vi "Check For Hardlink.vi"(8 "Error In":errorcluster, 10 "File Path":path, 11 "Configuration":T1) -> (0 "Error Out":errorcluster, 1 "Multiple Hardlinks":bool, 2 "Dup File Path":path, 3 "Configuration":T1)   [LabVIEW 2011, in "LVH-Toolbox.lvlib" / "LVH-Build-Tools.lvlib"]
uses:
  LVH-Build-Tools.lvlib
  Type Defs/Configuration.ctl
  Type Defs/Install Configuration.ctl
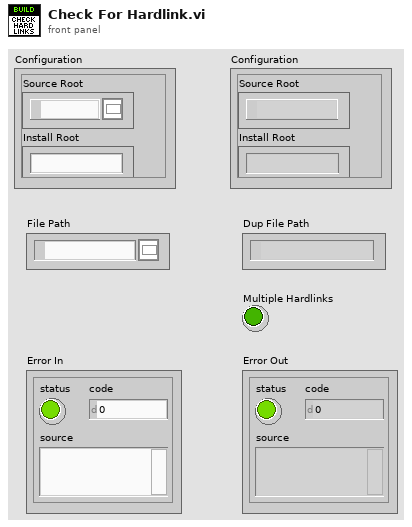
[diagram p1: front panel]
types:
  T1 = typedef "LVH-Toolbox.lvlib/LVH-Build-Tools.lvlib/Configuration.ctl" = cluster{"Source Root":path, "Install Root":string, "Components":string[], "Ignore":string[], "Config Files":path[], "LV Directories":path[], "Install Paths":T2}
  T2 = typedef "LVH-Toolbox.lvlib/LVH-Build-Tools.lvlib/Install Configuration.ctl" = cluster{"LabVIEW Directory":path, "Project Source Config":path}
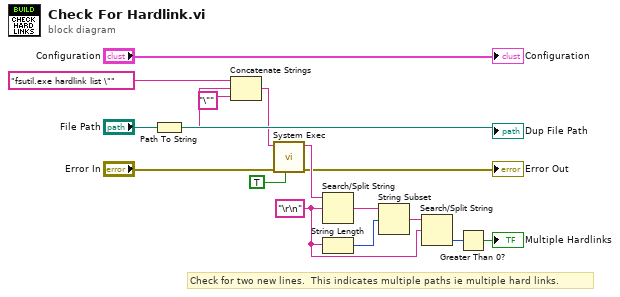
[diagram p0: block diagram]
diagram:
  w5 = "\r\n" ("search string/char (-)")
  # "Check for two new lines.  This indicates multiple paths ie multiple hard links."
  n1 = Path To String(path="File Path") -> (string=w14:string)
  n2 = Concatenate Strings("fsutil.exe hardlink list \"", w14, "\"" ("string")) -> (w13:string)
  n3 = call <vilib>:"System Exec.vi"("run minimized? (F)"=TRUE, "error in (no error)"="Error In", "command line"=w13) -> ("error out"=→"Error Out":errorcluster, "standard output"=w10:string)  [unwired: 5 in, 2 out]
  n4 = Search/Split String(string=w10, search string/char (-)=w5) -> (match + rest of string=w4:string)  [unwired: 1 in, 2 out]
  n5 = String Length(string=w5) -> (length=w6:i32)
  n6 = String Subset(string=w4, offset (0)=w6) -> (substring=w3:string)  [unwired: 1 in]
  n7 = Search/Split String(string=w3, search string/char (-)=w5) -> (offset of match=w8:i32)  [unwired: 1 in, 2 out]
  n8 = Greater Than 0?(x=w8) -> (x > 0?=→"Multiple Hardlinks":bool)
  "Configuration" <- "Configuration"
  "Dup File Path" <- "File Path"
